vi "Main.vi"() -> ()   [LabVIEW 2013]
uses:
  source_vi/gui/type_def/device_array.ctl
  source_vi/gui/type_def/device.ctl
  source_vi/gui/type_def/general.ctl
  source_vi/gui/type_def/general_and_device.ctl
  source_vi/queues/que_enqueue_message_single.vi
  source_vi/gui/global_var.vi
panel:
  out "Application:Command Line Arguments":string[](array[string])
  out "2DArray":string[][](array[string])
  in  "config_files":string(combo) caption="Configuration file"
  out "log_bar":cluster{u8, u8}(slide) caption="Logging" scale=10.0..100.0
  out "srv_bar":cluster{u8, u8}(slide) caption="Server" scale=10.0..100.0
  in  "logging?":bool
  in  "gral_&-device":T1={"general"={"file_ext"="0.0.0.0", "TCP port"=0, "#devices"=0, "log?"=FALSE, "tcp?"=FALSE, "language"="ENG"}, "eeg_device"={"name"="", "hardware"="", "image"=path "", "path"=path "", "extra"="", "channels"=""}}
  out "eeg_device":T3
  in  "serving?":bool
  in  "acquiring?":bool
  in  "stopBars":bool
  out "acq_bar":cluster{u8, u8}(slide) caption="Acquistion" scale=10.0..100.0
  in  "log?":bool caption="Save Log"
  in  "tcp?":bool caption="Save Log"
  in  "refuse mrk?":bool
  out "images":picture[](array[picture])
  out "general":T2={"file_ext"="CSV", "TCP port"=0, "#devices"=0, "log?"=FALSE, "tcp?"=FALSE, "language"="ENG"}
  out "devices":T4
  in  "play?":bool
  out "log_box":string
  in  "stop?":bool
  in  "eeg_txtbox":string(combo) caption="Device"
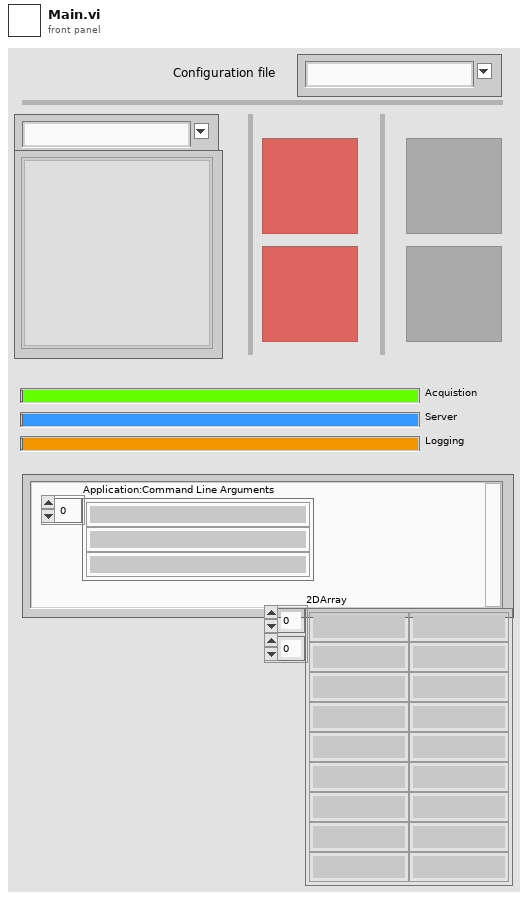
[diagram p1: front panel]
types:
  T1 = typedef "general_and_device.ctl" = cluster{"general":T2, "eeg_device":T3}
  T2 = typedef "general.ctl" = cluster{"file_ext":string, "TCP port":i32, "#devices":i32, "log?":bool, "tcp?":bool, "language":string}
  T3 = typedef "device.ctl" = cluster{"name":string, "hardware":string, "image":path, "path":path, "extra":string, "channels":string}
  T4 = typedef "device_array.ctl" = T3[]
  T5 = typedef "que_all_message_queues.ctl" = cluster{"UI":refnum<queue>, "Acquisition":refnum<queue>, "Server":refnum<queue>, "Logging":refnum<queue>}
  T6 = typedef "imagedata.ctl" = cluster{"image type":i32, "image depth":i32, "image":u8[], "mask":u8[], "colors":u32[], "Rectangle":cluster{"left":i16, "top":i16, "right":i16, "bottom":i16}}
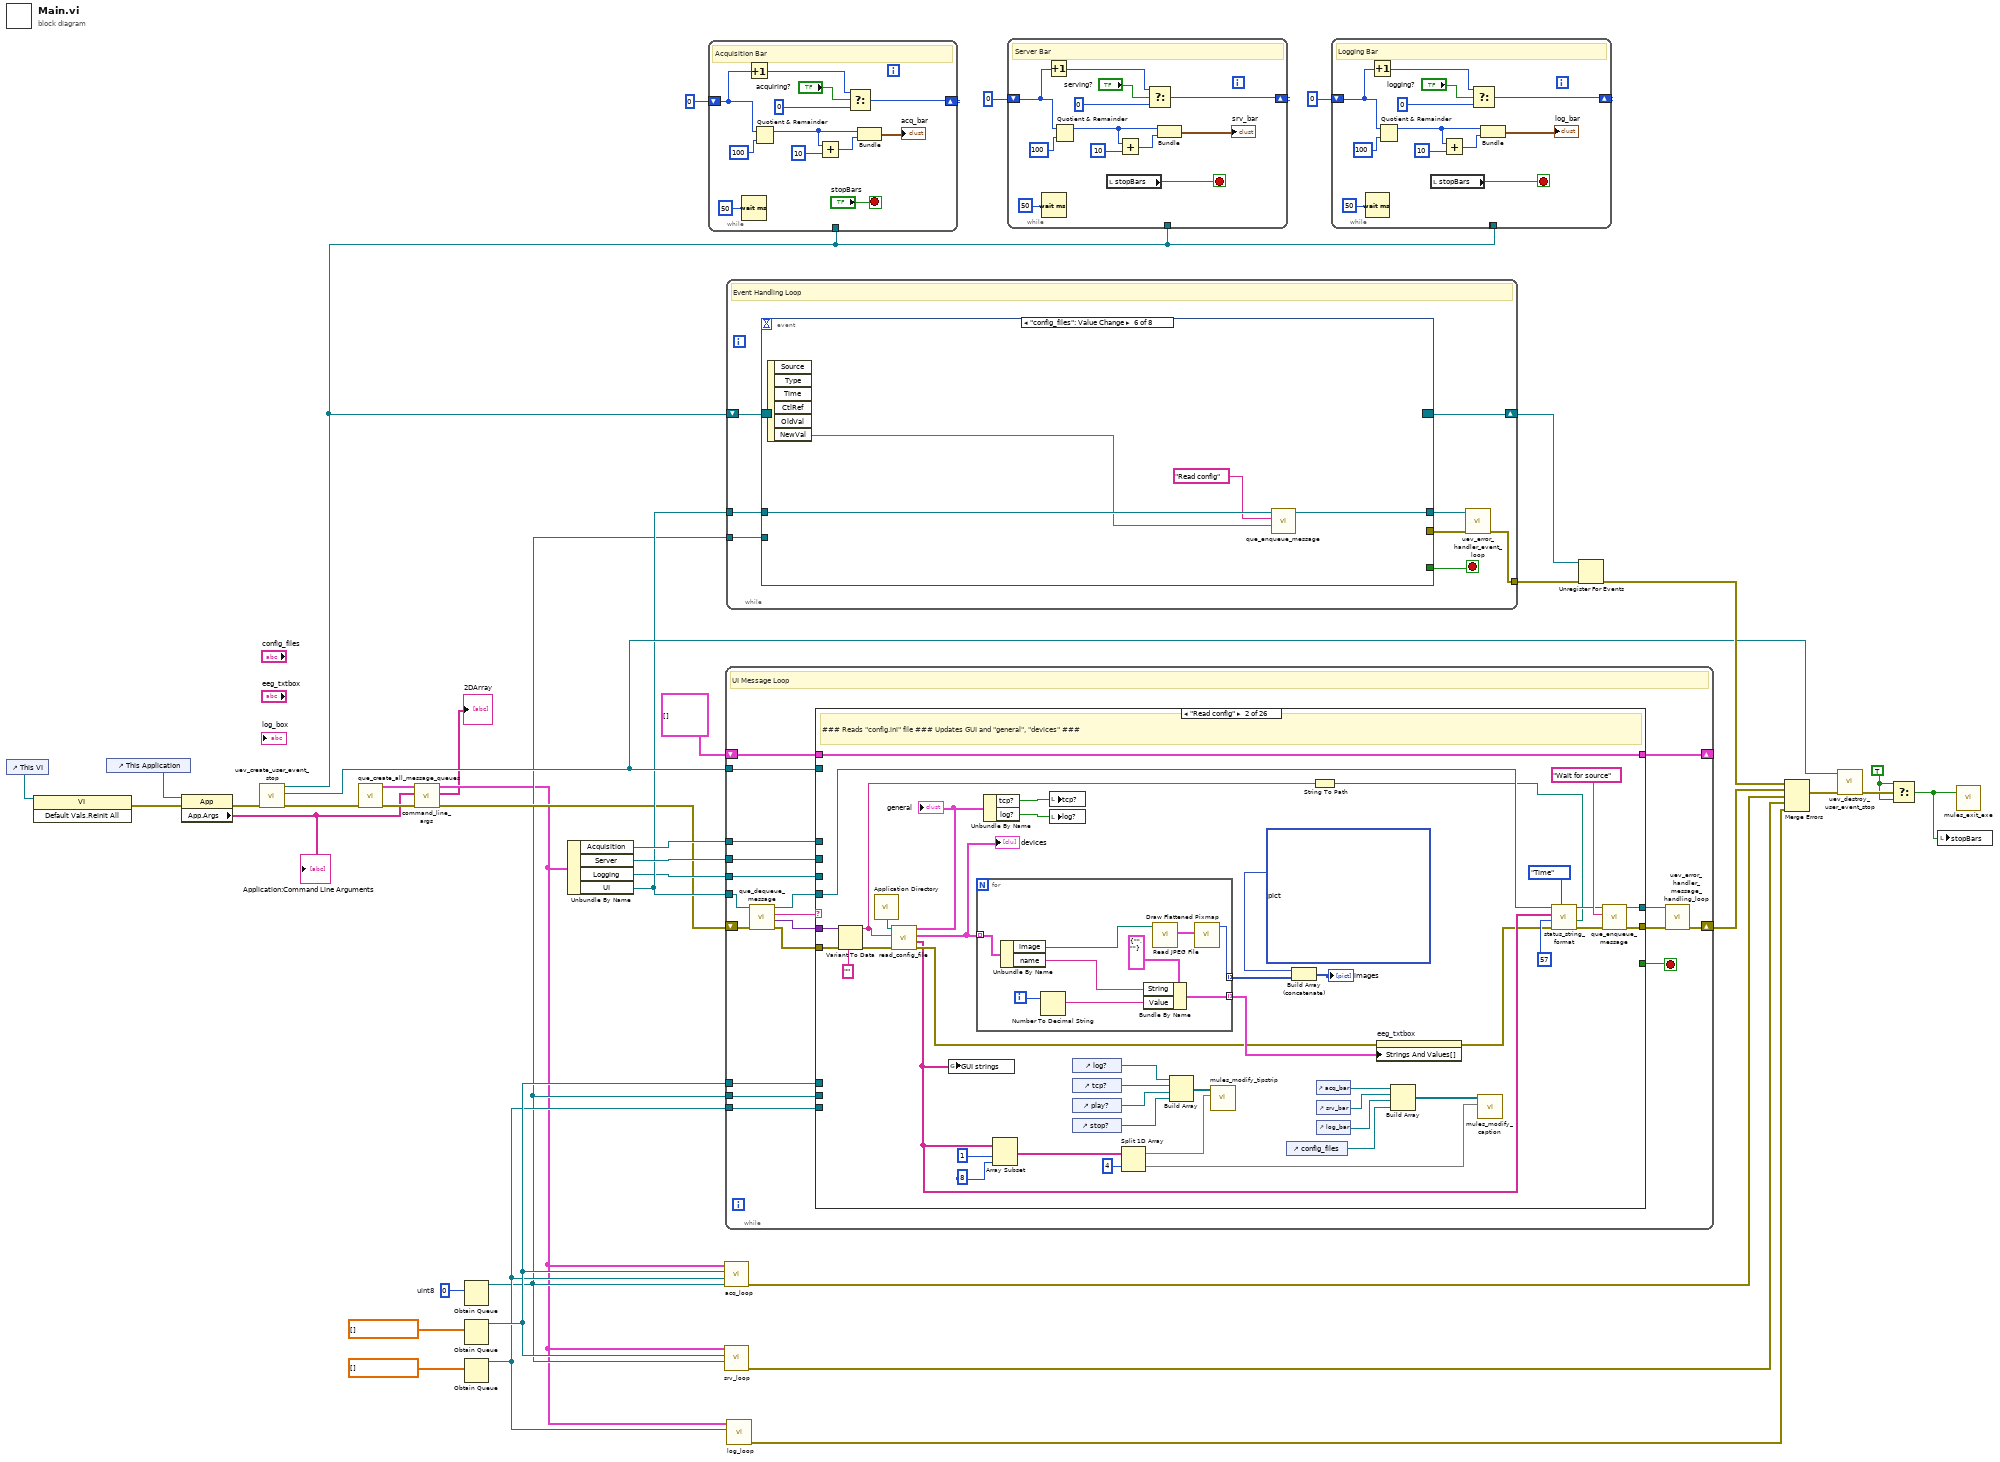
[diagram p0: block diagram]
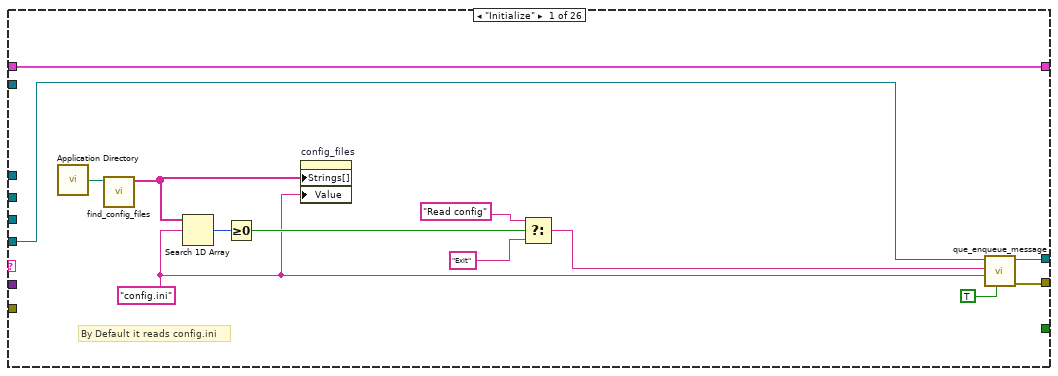
[diagram p2: hidden frame]
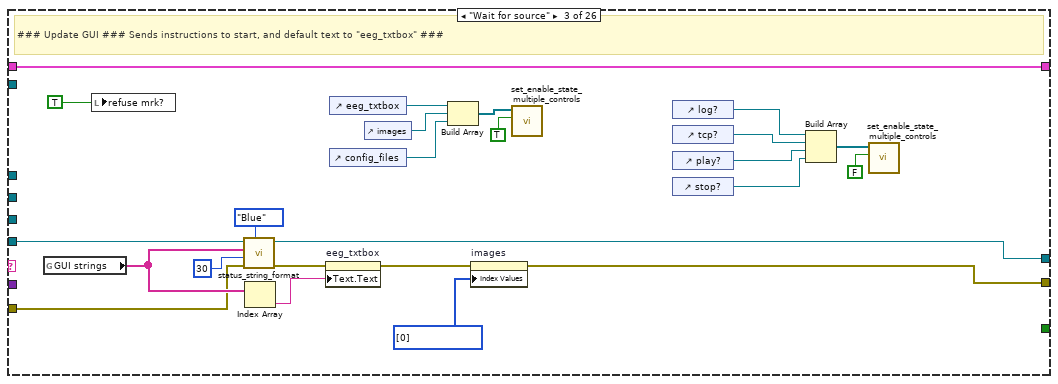
[diagram p3: hidden frame]
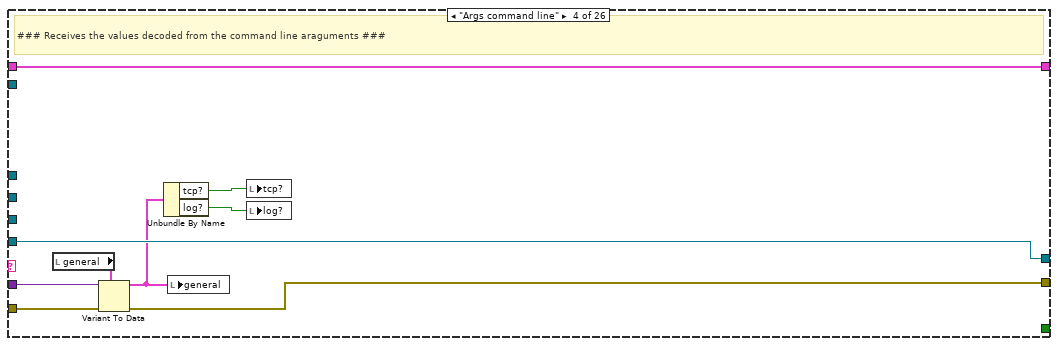
[diagram p4: hidden frame]
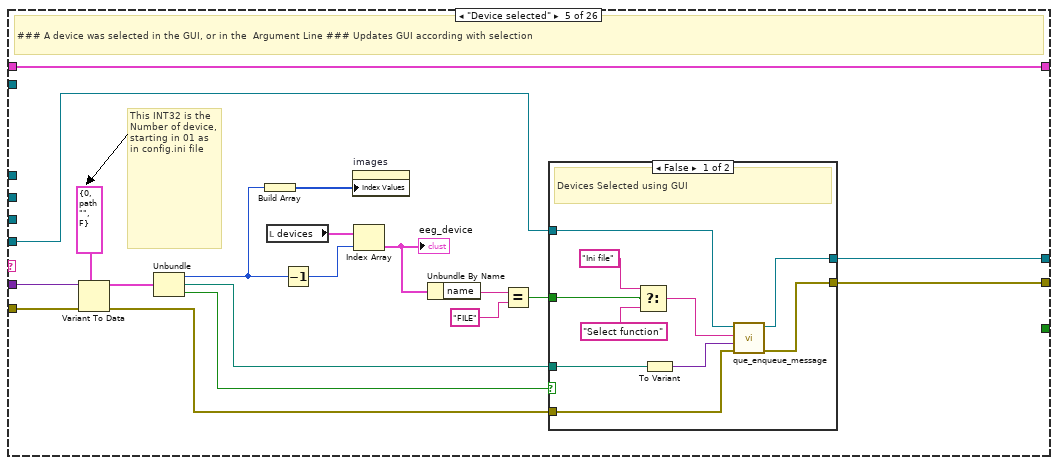
[diagram p5: hidden frame]
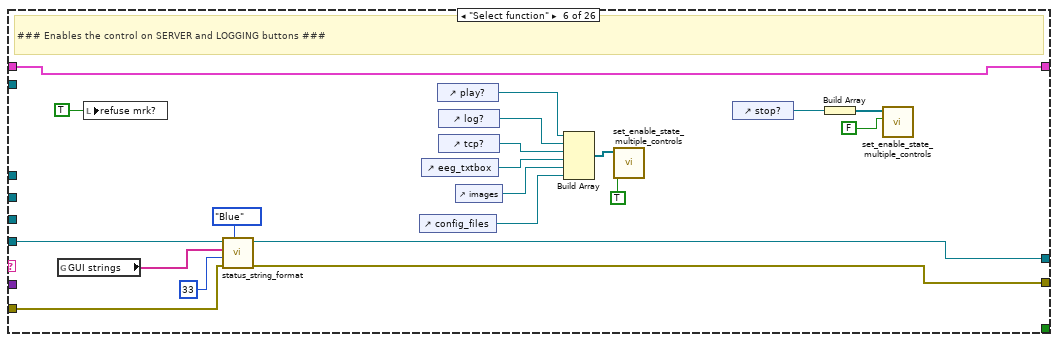
[diagram p7: hidden frame]
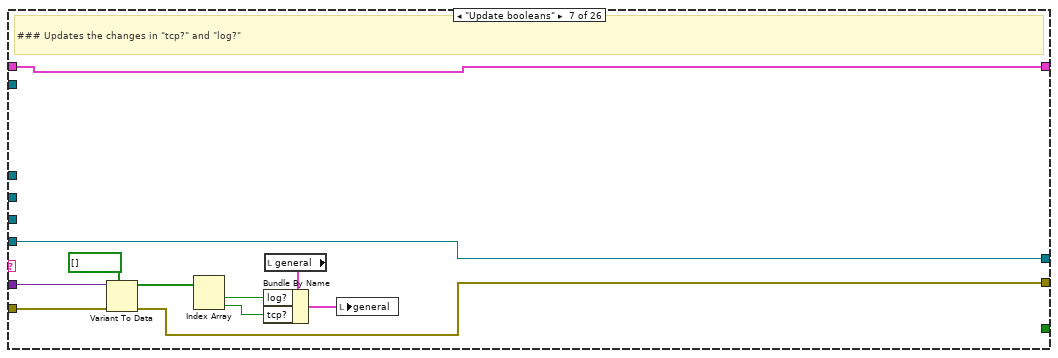
[diagram p8: hidden frame]
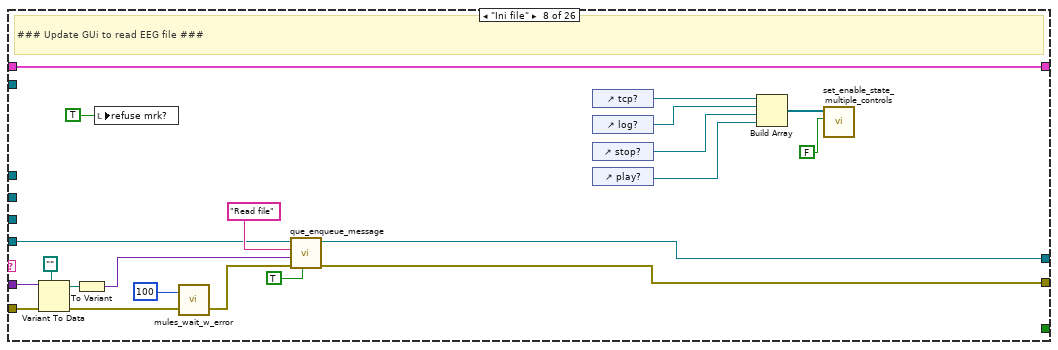
[diagram p9: hidden frame]
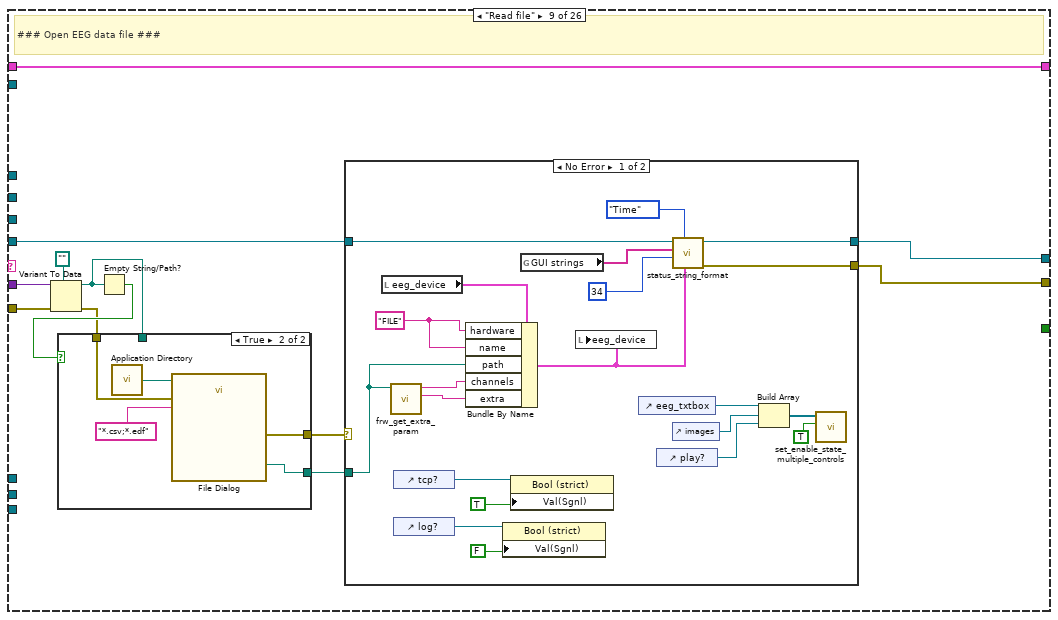
[diagram p10: hidden frame]
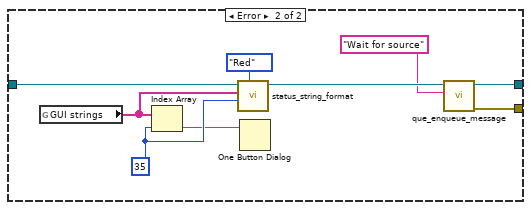
[diagram p12: hidden frame]
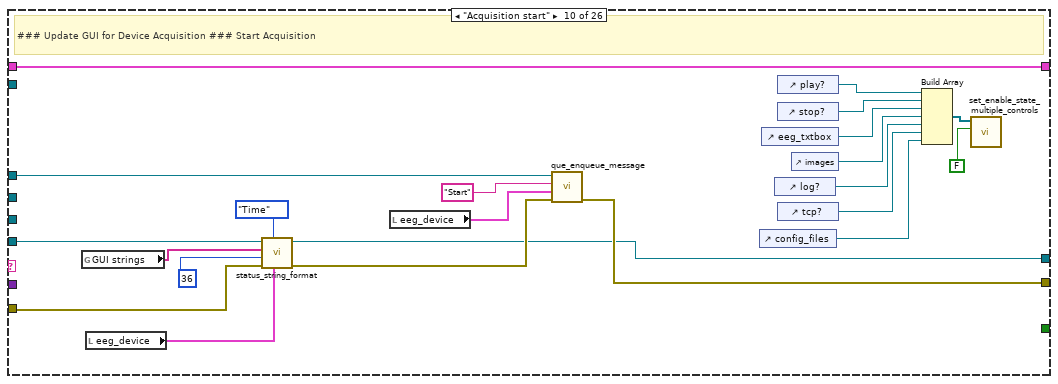
[diagram p13: hidden frame]
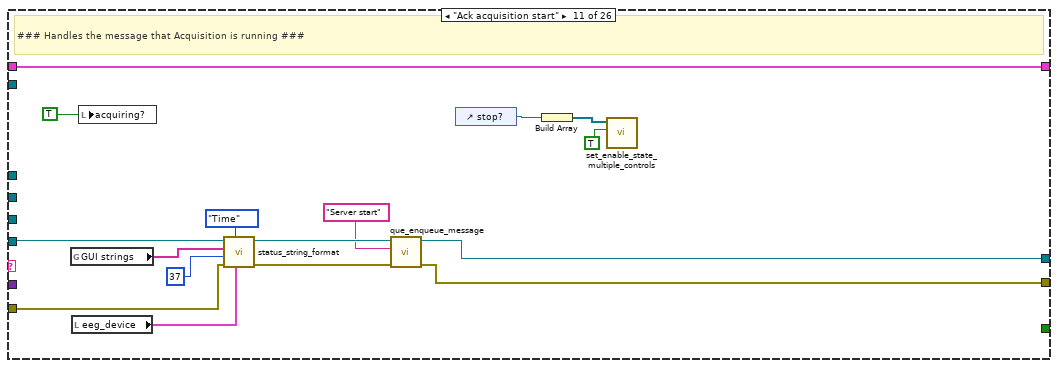
[diagram p14: hidden frame]
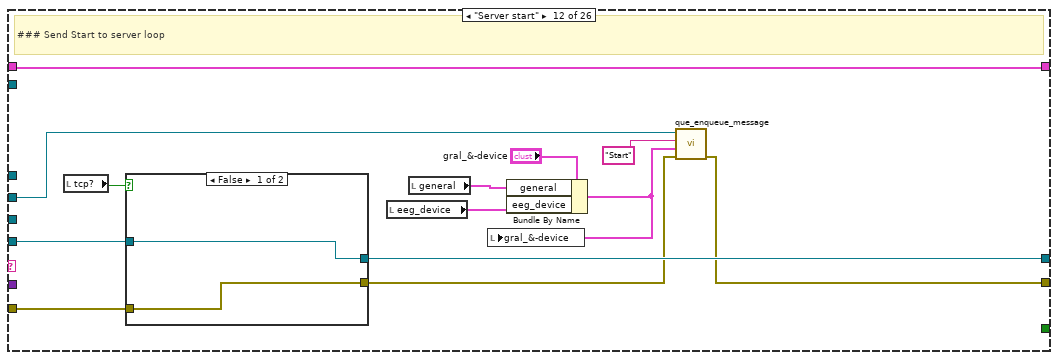
[diagram p15: hidden frame]
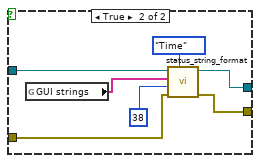
[diagram p16: hidden frame]
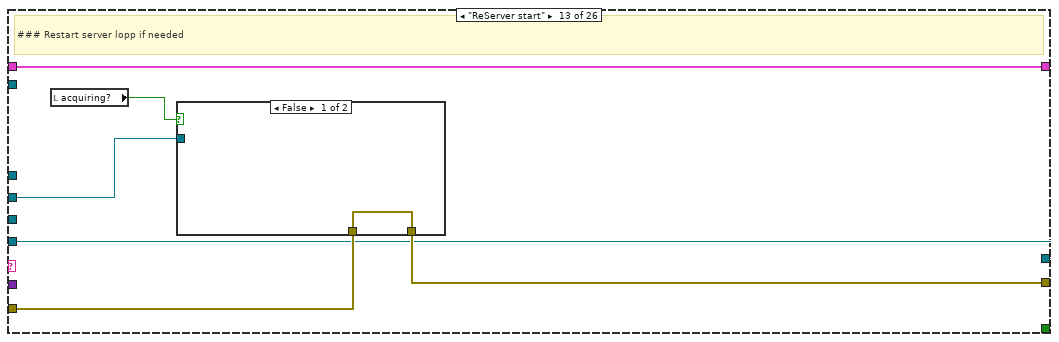
[diagram p17: hidden frame]
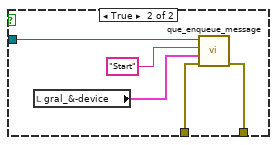
[diagram p18: hidden frame]
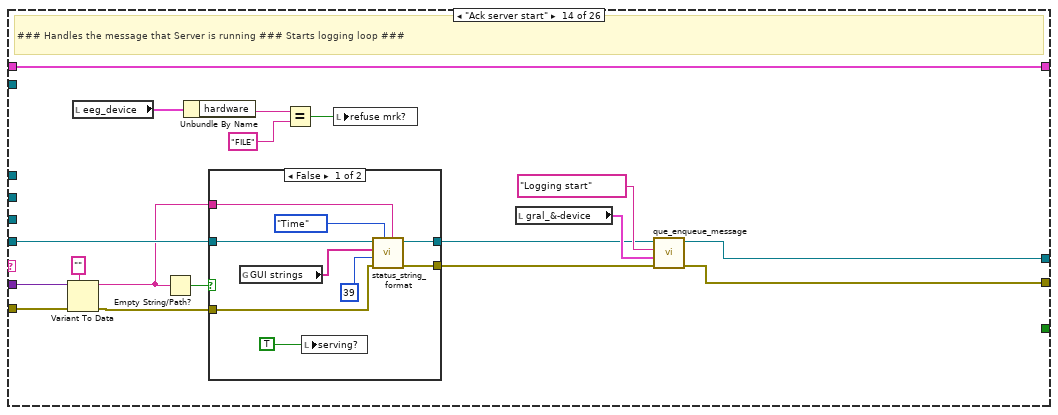
[diagram p19: hidden frame]
diagram:
  w22 = TRUE
  w29 = u8 0  # uint8
  n1 = control-ref of="This VI"() -> (w30:refnum<vi>)
  n2 = invoke class="VI" method="Default Vals.Reinit All"(reference=w30) -> (error out=w12:errorcluster)  [unwired: 2 in, 2 out]
  n3 = control-ref of="This Application"() -> (w14:refnum<vi>)
  n4 = property class="App"(reference=w14, error in=w12) -> (error out=w13:errorcluster, "App.Args"=w8:string[])  [unwired: 1 out]
  "Application:Command Line Arguments" <- w8
  n5 = call "uev_create_user_event_stop.vi"("error in (no error)"=w13) -> ("error out"=w25:errorcluster, "User Event - Stop"=w33:refnum<user-event>, "Stop Event Registration Refnum"=w6:refnum<event-registration>)  [unwired: 8 in]
  n6 = call "que_create_all_message_queues.vi"("error in (no error)"=w25) -> ("error out"=w10:errorcluster, "Message Queues out"=w9:T5)  [unwired: 9 in]
  n7 = call "command_line_args.vi"("error in (no error)"=w10, "App.Args"=w8, "Message Queues In"=w9) -> ("error out"=w11:errorcluster, "2D Array"=→"2DArray":string[][], "Message Queues Out"=w2:T5)  [unwired: 6 in]
  n8 = Obtain Queue(element data type=w29) -> (queue out=w3:refnum<queue>)  [unwired: 4 in, 2 out]
  n9 = Obtain Queue(element data type=dbl[] []) -> (queue out=w18:refnum<queue>)  [unwired: 4 in, 2 out]
  n10 = Obtain Queue(element data type=dbl[] []) -> (queue out=w4:refnum<queue>)  [unwired: 4 in, 2 out]
  n11 = Unbundle By Name(w2) -> ("Acquisition"=w32:refnum<queue>, "Server"=w31:refnum<queue>, "Logging"=w20:refnum<queue>, "UI"=w21:refnum<queue>)
  n12 = while {
    shift-right: [w42] -> _
    shift-left: 0 ("y") -> [w44]
    tunnel: w6 -> [_]
    stop <- "stopBars" stop-if-true
    # "Acquisition Bar"
    n13 = Wait (ms)(milliseconds to wait=u32 50 ("millisecond multiple")) -> ()  [unwired: 1 out]
    n14 = Increment(x=w44) -> (x+1=w43:i32)
    n15 = Quotient & Remainder(x=w44, y=100) -> (x-y*floor(x/y)=w47:i32)  [unwired: 1 out]
    n16 = Add(x=w47, y=u32 10 ("millisecond multiple")) -> (x+y=w50:u32)
    n17 = Select(t=w43, s="acquiring?", f=0 ("y")) -> (s? t:f=w42:i32)
    n18 = Bundle(w47, w50) -> (→"acq_bar":cluster{i32, u32})  [unwired: 1 in]
  }
  n19 = call "acq_loop.vi"("Marker Queue"=w3, "Log queue"=w4, "Server queue"=w18, "Message Queues"=w2) -> ("error out"=w24:errorcluster)  [unwired: 7 in]
  n20 = call "srv_loop.vi"("Marker Queue"=w3, "Server queue"=w18, "Message Queues"=w2) -> ("error out"=w19:errorcluster)  [unwired: 8 in]
  n21 = while {
    tunnel: w21 -> [w68]
    shift-right: [w56] -> w34
    shift-left: w11 -> [w69]
    tunnel: w31 -> [w63]
    tunnel: w33 -> [w62]
    tunnel: w32 -> [w61]
    tunnel: w18 -> [w54]
    tunnel: w3 -> [w59]
    shift-right: [w57] -> _
    shift-left: cluster{"String":string, "Color Box":u32}[] [] -> [w58]
    tunnel: w20 -> [w55]
    tunnel: w4 -> [w52]
    stop <- w60 stop-if-true
    # "UI Message Loop"
    n22 = call "que_dequeue_message.vi"("error in (no error)"=w69, "Message Queue"=w68) -> ("error out"=w67:errorcluster, "Message Data"=w66:variant, "Message"=w51:string, "dup Message Queue"=w65:refnum<queue>)  [unwired: 6 in]
    n23 = case shown="\"Read config\"" w51 {
      selector: w51 -> [_ _ _ _ _ _ _ _ _ _ _ _ _ _ _ _ _ _ _ _ _ _ _ _ _ w702]
      tunnel: w67 -> [_ w97 w137 w164 w168 w202 w221 w235 w252 w315 w327 w342 w363 w386 w404 w415 w438 w456 w485 w508 w532 w558 w607 w666 w693 w714]
      tunnel: w66 -> [_ w98 _ w167 w181 _ w227 w236 w255 _ _ _ _ w388 _ w416 w436 w459 w484 w512 w531 w560 w622 _ w692 _]
      tunnel: w65 -> [w77 w90 w156 w162 w178 w209 w219 w238 w262 w320 w333 w345 w361 w385 w402 w412 w444 w453 w477 w509 w528 w550 _ w663 w691 w715]
      tunnel: [w82 w93 w140 w163 w177 w201 w220 w240 w257 w310 w329 w338 w362 w379 w403 w411 w440 w461 w487 w506 w530 w548 w608 w665 w690 w703] -> w64
      tunnel: w63 -> [_ _ _ _ _ _ _ _ _ _ _ w341 w364 _ _ _ _ _ w488 _ _ _ _ _ _ w712]
      tunnel: w62 -> [_ _ _ _ _ _ _ _ _ _ _ _ _ _ _ _ _ _ _ _ _ _ _ _ _ w713]
      tunnel: w61 -> [_ _ _ _ _ _ _ _ _ w312 _ _ _ _ _ _ w442 _ _ _ _ w547 _ _ _ w711]
      tunnel: [_ _ _ _ _ _ _ _ _ _ _ _ _ _ _ _ _ _ _ _ _ _ _ _ _ TRUE ("Discard?")] -> w60
      tunnel: w54 -> [_ _ _ _ _ _ _ _ _ _ _ _ _ _ _ _ _ _ _ _ _ _ _ _ _ w708]
      tunnel: w59 -> [_ _ _ _ _ _ _ _ _ _ _ _ _ _ _ _ _ _ _ _ _ _ _ _ _ w707]
      tunnel: w58 -> [w80 w118 w139 w165 w172 w214 w222 w245 w261 w321 w323 w350 w365 w389 w401 w409 w449 w475 w490 w513 w537 w559 w620 w669 w689 w700]
      tunnel: [w80 w118 w139 w165 w172 w214 w222 w245 w261 w321 w323 w350 w365 w389 w401 w409 w449 w475 w490 w513 w537 w559 w613 w669 w689 w700] -> w57
      tunnel: w55 -> [_ _ _ _ _ _ _ _ _ _ _ _ _ _ w405 _ _ _ _ _ w524 _ _ _ _ w701]
      tunnel: [w81 w92 w136 w162 w176 w200 w219 w239 w258 w309 w328 w343 w361 w372 w402 w410 w443 w457 w478 w505 w525 w549 _ w664 w686 _] -> w53
      tunnel: w52 -> [_ _ _ _ _ _ _ _ _ _ _ _ _ _ _ _ _ _ _ _ _ _ _ _ _ w704]
      frame "Initialize" {
        w72 = "config.ini" ("Message")
        # "By Default it reads config.ini"
        n24 = call <vilib>:"Application Directory.vi"() -> ("Application Directory"=w78:path)
        n25 = call "find_config_files.vi"("path"=w78) -> ("config files_names"=w75:string[])  [unwired: 10 in]
        n26 = Search 1D Array(1D array=w75, element=w72) -> (index of element=w76:i32)  [unwired: 1 in]
        n27 = Greater Or Equal To 0?(x=w76) -> (x >= 0?=w73:bool)
        n28 = property on="config_files" class="CmbBox"("Strings[]"=w75, "Value"=w72) -> ()  [unwired: 2 in, 2 out]
        n29 = Select(t="Read config" ("Message"), s=w73, f="Exit" ("Message")) -> (s? t:f=w74:string)
        n30 = call-poly "que_enqueue_message.vi"("Priority Message? (F)"=TRUE, "Message Data"=w72, "Message"=w74, "Message Queue"=w77) -> ("error out"=w82:errorcluster, "dup Message Queue"=w81:refnum<queue>)  [unwired: 6 in]
      }
      frame "Read config" {
        # "### Reads \"config.ini\" file ### Updates GUI and \"general\", \"devices\" ###"
        n31 = Variant To Data(error in=w97, type="", Variant=w98) -> (data=w87:string, error out=w96:errorcluster)
        n32 = call <vilib>:"Application Directory.vi"() -> ("Application Directory"=w100:path)
        n33 = call "read_config_file.vi"("error in (no error)"=w96, "filename"=w87, "Application Directory"=w100) -> ("error out"=w117:errorcluster, "gui_strings"=w88:string[], "devices"=w119:T4, "gral_config"=w125:T2)  [unwired: 5 in]
        "devices" <- w119
        "general" <- w125
        n34 = global write "global_var.vi" "GUI strings"(w88) -> ()
        n35 = for {
          tunnel: w119 -> [w134] mode=indexing
          tunnel: [w132] -> w123 mode=indexing
          tunnel: [w128] -> w124 mode=indexing
          i -> [w131]
          n36 = Unbundle By Name(w134) -> ("image"=w126:path, "name"=w127:string)
          n37 = Number To Decimal String(number=w131) -> (decimal integer string=w129:string)  [unwired: 1 in]
          n38 = Bundle By Name(cluster=cluster{"String":string, "Value":string} {"String"="", "Value"=""} ("element"), "String"=w127, "Value"=w129) -> (w128:cluster{"String":string, "Value":string})
          n39 = call <vilib>:"Read JPEG File.vi"("path to JPEG file"=w126) -> ("image data"=w133:T6)  [unwired: 8 in, 2 out]
          n40 = call <vilib>:"Draw Flattened Pixmap.vi"("image data"=w133) -> ("new picture"=w132:picture)  [unwired: 8 in]
        }
        n41 = Unbundle By Name(w125) -> ("tcp?"=w121:bool, "log?"=w120:bool)
        n42 = Array Subset(array=w88, index=1, length=8) -> (w105:string[])
        n43 = local write "tcp?"(w121) -> ()
        n44 = local write "log?"(w120) -> ()
        n45 = control-ref of="log?"() -> (w114:refnum<vi>)
        n46 = control-ref of="tcp?"() -> (w113:refnum<vi>)
        n47 = control-ref of="play?"() -> (w112:refnum<vi>)
        n48 = control-ref of="stop?"() -> (w111:refnum<vi>)
        n49 = Split 1D Array(array=w105, index=4) -> (first subarray=w103:string[], second subarray=w102:string[])
        n50 = Build Array(w114, w113, w112, w111) -> (w110:refnum<vi>[])
        n51 = call "mules_modify_tipstrip.vi"("Tip Strip Array"=w103, "Controls"=w110) -> ()  [unwired: 10 in]
        n52 = control-ref of="config_files"() -> (w95:refnum<vi>)
        n53 = Build Array (concatenate)(picture bytes[110622] ("2D Picture"), w123) -> (→"images":picture[])
        n54 = String To Path(string=w87) -> (path=w86:path)
        n55 = control-ref of="acq_bar"() -> (w109:refnum<vi>)
        n56 = control-ref of="srv_bar"() -> (w108:refnum<vi>)
        n57 = control-ref of="log_bar"() -> (w107:refnum<vi>)
        n58 = property on="eeg_txtbox" class="CmbBox"(error in=w117, "Strings And Values[]"=w124) -> (error out=w83:errorcluster)  [unwired: 1 in, 1 out]
        n59 = Build Array(w109, w108, w107, w95) -> (w106:refnum<vi>[])
        n60 = call "mules_modify_caption.vi"("Tip Strip Array"=w102, "Controls"=w106) -> ()  [unwired: 10 in]
        n61 = call "status_string_format.vi"("log_file"=w86, "color"=enum16{"Black", "Blue", "Red", "Time"}."Time", "error in (no error)"=w83, "index"=57, "gui_strings"=w88, "Message Queue"=w90) -> ("error out"=w89:errorcluster, "dup Message Queue"=w91:refnum<queue>)  [unwired: 4 in]
        n62 = call-poly "que_enqueue_message.vi"("error in (no error)"=w89, "Message"="Wait for source", "Message Queue"=w91) -> ("error out"=w93:errorcluster, "dup Message Queue"=w92:refnum<queue>)  [unwired: 7 in]
      }
      frame "Wait for source" {
        # "### Update GUI ### Sends instructions to start, and default text to \"eeg_txtbox\" ###"
        n63 = global read "global_var.vi" "GUI strings"() -> (w138:string[])
        n64 = local write "refuse mrk?"(TRUE) -> ()
        n65 = call "status_string_format.vi"("color"=enum16{"Black", "Blue", "Red", "Time"}."Blue", "error in (no error)"=w137, "index"=30, "gui_strings"=w138, "Message Queue"=w156) -> ("error out"=w152:errorcluster, "dup Message Queue"=w136:refnum<queue>)  [unwired: 5 in]
        n66 = Index Array(array=w138) -> (element=w153:string)  [unwired: 1 in]
        n67 = property on="eeg_txtbox" class="CmbBox"(error in=w152, "Text.Text"=w153) -> (error out=w155:errorcluster)  [unwired: 1 in, 1 out]
        n68 = control-ref of="eeg_txtbox"() -> (w144:refnum<vi>)
        n69 = control-ref of="config_files"() -> (w135:refnum<vi>)
        n70 = control-ref of="images"() -> (w143:refnum<vi>)
        n71 = Build Array(w144, w143, w135) -> (w141:refnum<vi>[])
        n72 = property on="images" class="Arr (strict)"(error in=w155, "Index Values"=u32[] [0]) -> (error out=w140:errorcluster)  [unwired: 1 in, 1 out]
        n73 = call "set_enable_state_multiple_controls.vi"("Enable?"=TRUE, "Controls"=w141) -> ()  [unwired: 10 in]
        n74 = control-ref of="log?"() -> (w145:refnum<vi>)
        n75 = control-ref of="tcp?"() -> (w146:refnum<vi>)
        n76 = control-ref of="play?"() -> (w147:refnum<vi>)
        n77 = control-ref of="stop?"() -> (w148:refnum<vi>)
        n78 = Build Array(w145, w146, w147, w148) -> (w151:refnum<vi>[])
        n79 = call "set_enable_state_multiple_controls.vi"("Enable?"=FALSE, "Controls"=w151) -> ()  [unwired: 10 in]
      }
      frame "Args command line" {
        # "### Receives the values decoded from the command line araguments ###"
        n80 = local read "general"() -> (w166:T2)
        n81 = Variant To Data(error in=w164, type=w166, Variant=w167) -> (data=w159:T2, error out=w163:errorcluster)
        n82 = Unbundle By Name(w159) -> ("tcp?"=w161:bool, "log?"=w160:bool)
        n83 = local write "general"(w159) -> ()
        n84 = local write "tcp?"(w161) -> ()
        n85 = local write "log?"(w160) -> ()
      }
      frame "Device selected" {
        # "This INT32 is the Number of device, starting in 01 as in config.ini file"
        # "### A device was selected in the GUI, or in the  Argument Line ### Updates GUI according with selection"
        n86 = Variant To Data(error in=w168, type=cluster{i32, path, bool} {0, path "", FALSE} ("output cluster"), Variant=w181) -> (data=w175:cluster{i32, path, bool}, error out=w169:errorcluster)
        n87 = Unbundle(w175) -> (w174:i32, w173:path, w170:bool)
        n88 = Build Array(w174) -> (w180:i32[])
        n89 = local read "devices"() -> (w182:T4)
        n90 = Decrement(x=w174) -> (x-1=w179:i32)
        n91 = property on="images" class="Arr (strict)"("Index Values"=w180) -> ()  [unwired: 2 in, 2 out]
        n92 = Index Array(array=w182, index=w179) -> (element=w183:T3)
        "eeg_device" <- w183
        n93 = Unbundle By Name(w183) -> ("name"=w184:string)
        n94 = Equal?(x=w184, y="FILE" ("Message")) -> (x = y?=w186:bool)
        n95 = case shown="False" w170 {
          tunnel: w186 -> [w193 _]
          tunnel: w178 -> [w192 w198]
          tunnel: [w191 w197] -> w177
          tunnel: [w190 w198] -> w176
          tunnel: w173 -> [w189 _]
          tunnel: w169 -> [w187 w197]
          frame False {
            # "Devices Selected using GUI"
            n96 = Select(t="Ini file" ("Message"), s=w193, f="Select function" ("Message")) -> (s? t:f=w196:string)
            n97 = To Variant(anything=w189) -> (Variant=w188:variant)
            n98 = call-poly "que_enqueue_message.vi"("error in (no error)"=w187, "Message Data"=w188, "Message"=w196, "Message Queue"=w192) -> ("error out"=w191:errorcluster, "dup Message Queue"=w190:refnum<queue>)  [unwired: 6 in]
          }
          frame True {
            # "Device Selected in Argument Line"
          }
        }
      }
      frame "Select function" {
        # "### Enables the control on SERVER and LOGGING buttons ###"
        n99 = global read "global_var.vi" "GUI strings"() -> (w208:string[])
        n100 = local write "refuse mrk?"(TRUE) -> ()
        n101 = call "status_string_format.vi"("color"=enum16{"Black", "Blue", "Red", "Time"}."Blue", "error in (no error)"=w202, "index"=33, "gui_strings"=w208, "Message Queue"=w209) -> ("error out"=w201:errorcluster, "dup Message Queue"=w200:refnum<queue>)  [unwired: 5 in]
        n102 = control-ref of="config_files"() -> (w199:refnum<vi>)
        n103 = control-ref of="eeg_txtbox"() -> (w211:refnum<vi>)
        n104 = control-ref of="play?"() -> (w203:refnum<vi>)
        n105 = control-ref of="log?"() -> (w204:refnum<vi>)
        n106 = control-ref of="tcp?"() -> (w205:refnum<vi>)
        n107 = control-ref of="images"() -> (w210:refnum<vi>)
        n108 = Build Array(w203, w204, w205, w211, w210, w199) -> (w213:refnum<vi>[])
        n109 = call "set_enable_state_multiple_controls.vi"("Enable?"=TRUE, "Controls"=w213) -> ()  [unwired: 10 in]
        n110 = control-ref of="stop?"() -> (w218:refnum<vi>)
        n111 = Build Array(w218) -> (w217:refnum<vi>[])
        n112 = call "set_enable_state_multiple_controls.vi"("Enable?"=FALSE, "Controls"=w217) -> ()  [unwired: 10 in]
      }
      frame "Update booleans" {
        # "### Updates the changes in \"tcp?\" and \"log?\""
        n113 = Variant To Data(error in=w221, type=bool[] [], Variant=w227) -> (data=w225:bool[], error out=w220:errorcluster)
        n114 = Index Array(array=w225) -> (element #1=w224:bool, element #2=w223:bool)  [unwired: 2 in]
        n115 = local read "general"() -> (w228:T2)
        n116 = Bundle By Name(cluster=w228, "log?"=w224, "tcp?"=w223) -> (w229:T2)
        n117 = local write "general"(w229) -> ()
      }
      frame "Ini file" {
        # "### Update GUi to read EEG file ###"
        n118 = Variant To Data(error in=w235, type=path "", Variant=w236) -> (data=w232:path, error out=w234:errorcluster)
        n119 = To Variant(anything=w232) -> (Variant=w231:variant)
        n120 = local write "refuse mrk?"(TRUE) -> ()
        n121 = call "mules_wait_w_error.vi"("error in (no error)"=w234, "milliseconds to wait"=u32 100) -> ("error out"=w242:errorcluster)  [unwired: 1 in]
        n122 = call-poly "que_enqueue_message.vi"("Priority Message? (F)"=TRUE, "error in (no error)"=w242, "Message Data"=w231, "Message"="Read file", "Message Queue"=w238) -> ("error out"=w240:errorcluster, "dup Message Queue"=w239:refnum<queue>)  [unwired: 5 in]
        n123 = control-ref of="tcp?"() -> (w237:refnum<vi>)
        n124 = control-ref of="log?"() -> (w244:refnum<vi>)
        n125 = control-ref of="stop?"() -> (w250:refnum<vi>)
        n126 = control-ref of="play?"() -> (w249:refnum<vi>)
        n127 = Build Array(w237, w244, w250, w249) -> (w248:refnum<vi>[])
        n128 = call "set_enable_state_multiple_controls.vi"("Enable?"=FALSE, "Controls"=w248) -> ()  [unwired: 10 in]
      }
      frame "Read file" {
        # "### Open EEG data file ###"
        n129 = Variant To Data(error in=w252, type=path "", Variant=w255) -> (data=w253:path, error out=w251:errorcluster)
        n130 = Empty String/Path?(string/path=w253) -> (empty?=w254:bool)
        n131 = case shown="True" w254 {
          tunnel: [w263 w269] -> w260
          tunnel: [w264 w268] -> w259
          tunnel: w253 -> [w264 _]
          tunnel: w251 -> [w263 w267]
          frame False {
          }
          frame True {
            n132 = call <vilib>:"Application Directory.vi"() -> ("Application Directory"=w265:path)
            n133 = call "File Dialog"("start path"=w265, "error in"=w267, "pattern (all files)"="*.csv;*.edf") -> ("selected path"=w268:path, "error out"=w269:errorcluster)  [unwired: 9 in, 2 out]
          }
        }
        n134 = case shown="No Error" w260 {
          tunnel: w262 -> [w286 w299]
          tunnel: w259 -> [w283 _]
          tunnel: [w287 w294] -> w258
          tunnel: [w279 w292] -> w257
          frame No Error {
            w280 = "FILE" ("Message")
            n135 = local read "eeg_device"() -> (w290:T3)
            n136 = call "frw_get_extra_param.vi"("Path"=w283) -> ("extra_string"=w281:string, "channels_str"=w282:string)  [unwired: 9 in]
            n137 = control-ref of="tcp?"() -> (w270:refnum<vi>)
            n138 = control-ref of="log?"() -> (w273:refnum<vi>)
            n139 = Bundle By Name(cluster=w290, "hardware"=w280, "name"=w280, "path"=w283, "channels"=w282, "extra"=w281) -> (w285:T3)
            n140 = property class="Bool (strict)"(reference=w273, "Val(Sgnl)"=FALSE ("Value (Signaling)")) -> ()  [unwired: 1 in, 2 out]
            n141 = property class="Bool (strict)"(reference=w270, "Val(Sgnl)"=TRUE ("Value (Signaling)")) -> ()  [unwired: 1 in, 2 out]
            n142 = global read "global_var.vi" "GUI strings"() -> (w289:string[])
            n143 = local write "eeg_device"(w285) -> ()
            n144 = control-ref of="eeg_txtbox"() -> (w275:refnum<vi>)
            n145 = control-ref of="play?"() -> (w277:refnum<vi>)
            n146 = call "status_string_format.vi"("eeg_device"=w285, "color"=enum16{"Black", "Blue", "Red", "Time"}."Time", "index"=34, "gui_strings"=w289, "Message Queue"=w286) -> ("error out"=w279:errorcluster, "dup Message Queue"=w287:refnum<queue>)  [unwired: 5 in]
            n147 = control-ref of="images"() -> (w274:refnum<vi>)
            n148 = Build Array(w275, w274, w277) -> (w276:refnum<vi>[])
            n149 = call "set_enable_state_multiple_controls.vi"("Enable?"=TRUE, "Controls"=w276) -> ()  [unwired: 10 in]
          }
          frame Error {
            w297 = 35 ("index")
            n150 = global read "global_var.vi" "GUI strings"() -> (w298:string[])
            n151 = Index Array(array=w298, index=w297) -> (element=w291:string)
            n152 = call "status_string_format.vi"("color"=enum16{"Black", "Blue", "Red", "Time"}."Red", "index"=w297, "gui_strings"=w298, "Message Queue"=w299) -> ("dup Message Queue"=w295:refnum<queue>)  [unwired: 6 in, 1 out]
            n153 = One Button Dialog(message=w291) -> ()  [unwired: 1 in, 1 out]
            n154 = call-poly "que_enqueue_message.vi"("Message"="Wait for source", "Message Queue"=w295) -> ("error out"=w292:errorcluster, "dup Message Queue"=w294:refnum<queue>)  [unwired: 8 in]
          }
        }
      }
      frame "Acquisition start" {
        # "### Update GUI for Device Acquisition ### Start Acquisition"
        n155 = global read "global_var.vi" "GUI strings"() -> (w319:string[])
        n156 = local read "eeg_device"() -> (w316:T3)
        n157 = call "status_string_format.vi"("eeg_device"=w316, "color"=enum16{"Black", "Blue", "Red", "Time"}."Time", "error in (no error)"=w315, "index"=36, "gui_strings"=w319, "Message Queue"=w320) -> ("error out"=w311:errorcluster, "dup Message Queue"=w309:refnum<queue>)  [unwired: 4 in]
        n158 = local read "eeg_device"() -> (w313:T3)
        n159 = call-poly "que_enqueue_message.vi"("error in (no error)"=w311, "Message Data"=w313, "Message"="Start", "Message Queue"=w312) -> ("error out"=w310:errorcluster)  [unwired: 6 in, 1 out]
        n160 = control-ref of="config_files"() -> (w300:refnum<vi>)
        n161 = control-ref of="eeg_txtbox"() -> (w304:refnum<vi>)
        n162 = control-ref of="log?"() -> (w302:refnum<vi>)
        n163 = control-ref of="play?"() -> (w308:refnum<vi>)
        n164 = control-ref of="stop?"() -> (w307:refnum<vi>)
        n165 = control-ref of="tcp?"() -> (w301:refnum<vi>)
        n166 = control-ref of="images"() -> (w303:refnum<vi>)
        n167 = Build Array(w308, w307, w304, w303, w302, w301, w300) -> (w306:refnum<vi>[])
        n168 = call "set_enable_state_multiple_controls.vi"("Enable?"=FALSE, "Controls"=w306) -> ()  [unwired: 10 in]
      }
      frame "Ack acquisition start" {
        # "### Handles the message that Acquisition is running ###"
        n169 = global read "global_var.vi" "GUI strings"() -> (w337:string[])
        n170 = local read "eeg_device"() -> (w334:T3)
        n171 = local write "acquiring?"(TRUE ("runBar1?")) -> ()
        n172 = call "status_string_format.vi"("eeg_device"=w334, "color"=enum16{"Black", "Blue", "Red", "Time"}."Time", "error in (no error)"=w327, "index"=37, "gui_strings"=w337, "Message Queue"=w333) -> ("error out"=w330:errorcluster, "dup Message Queue"=w332:refnum<queue>)  [unwired: 4 in]
        n173 = call-poly "que_enqueue_message.vi"("error in (no error)"=w330, "Message"="Server start", "Message Queue"=w332) -> ("error out"=w329:errorcluster, "dup Message Queue"=w328:refnum<queue>)  [unwired: 7 in]
        n174 = control-ref of="stop?"() -> (w326:refnum<vi>)
        n175 = Build Array(w326) -> (w325:refnum<vi>[])
        n176 = call "set_enable_state_multiple_controls.vi"("Enable?"=TRUE, "Controls"=w325) -> ()  [unwired: 10 in]
      }
      frame "Server start" {
        # "### Send Start to server loop"
        n177 = local read "tcp?"() -> (w344:bool)
        n178 = case shown="False" w344 {
          tunnel: w345 -> [w351 w356]
          tunnel: w342 -> [w352 w355]
          tunnel: [w351 w354] -> w343
          tunnel: [w352 w353] -> w339
          frame False {
          }
          frame True {
            n179 = global read "global_var.vi" "GUI strings"() -> (w358:string[])
            n180 = call "status_string_format.vi"("color"=enum16{"Black", "Blue", "Red", "Time"}."Time", "error in (no error)"=w355, "index"=38, "gui_strings"=w358, "Message Queue"=w356) -> ("error out"=w353:errorcluster, "dup Message Queue"=w354:refnum<queue>)  [unwired: 5 in]
          }
        }
        n181 = local read "eeg_device"() -> (w346:T3)
        n182 = local read "general"() -> (w347:T2)
        n183 = Bundle By Name(cluster="gral_&-device", "general"=w347, "eeg_device"=w346) -> (w340:T1)
        n184 = local write "gral_&-device"(w340) -> ()
        n185 = call-poly "que_enqueue_message.vi"("error in (no error)"=w339, "Message Data"=w340, "Message"="Start", "Message Queue"=w341) -> ("error out"=w338:errorcluster)  [unwired: 6 in, 1 out]
      }
      frame "ReServer start" {
        # "### Restart server lopp if needed"
        n186 = local read "acquiring?"() -> (w360:bool)
        n187 = case shown="False" w360 {
          tunnel: w364 -> [_ w370]
          tunnel: w363 -> [w366 w368]
          tunnel: [w366 w367] -> w362
          frame False {
          }
          frame True {
            n188 = local read "gral_&-device"() -> (w369:T1)
            n189 = call-poly "que_enqueue_message.vi"("error in (no error)"=w368, "Message Data"=w369, "Message"="Start", "Message Queue"=w370) -> ("error out"=w367:errorcluster)  [unwired: 6 in, 1 out]
          }
        }
      }
      frame "Ack server start" {
        # "### Handles the message that Server is running ### Starts logging loop ###"
        n190 = Variant To Data(error in=w386, type="" ("String"), Variant=w388) -> (data=w381:string, error out=w378:errorcluster)
        n191 = local read "eeg_device"() -> (w377:T3)
        n192 = Empty String/Path?(string/path=w381) -> (empty?=w382:bool)
        n193 = Unbundle By Name(w377) -> ("hardware"=w376:string)
        n194 = case shown="False" w382 {
          tunnel: w385 -> [w398 w399]
          tunnel: w381 -> [w394 _]
          tunnel: [w393 w400] -> w380
          tunnel: w378 -> [w392 w400]
          tunnel: [w391 w399] -> w373
          frame False {
            n195 = global read "global_var.vi" "GUI strings"() -> (w397:string[])
            n196 = local write "serving?"(TRUE ("runBar1?")) -> ()
            n197 = call "status_string_format.vi"("ip"=w394, "color"=enum16{"Black", "Blue", "Red", "Time"}."Time", "error in (no error)"=w392, "index"=39, "gui_strings"=w397, "Message Queue"=w398) -> ("error out"=w393:errorcluster, "dup Message Queue"=w391:refnum<queue>)  [unwired: 4 in]
          }
          frame True {
          }
        }
        n198 = Equal?(x=w376, y="FILE") -> (x = y?=w374:bool)
        n199 = local write "refuse mrk?"(w374) -> ()
        n200 = local read "gral_&-device"() -> (w383:T1)
        n201 = call-poly "que_enqueue_message.vi"("error in (no error)"=w380, "Message Data"=w383, "Message"="Logging start", "Message Queue"=w373) -> ("error out"=w379:errorcluster, "dup Message Queue"=w372:refnum<queue>)  [unwired: 6 in]
      }
      frame "Logging start" {
        n202 = local read "gral_&-device"() -> (w406:T1)
        n203 = call-poly "que_enqueue_message.vi"("error in (no error)"=w404, "Message Data"=w406, "Message"="Start", "Message Queue"=w405) -> ("error out"=w403:errorcluster)  [unwired: 6 in, 1 out]
      }
      frame "Ack logging start" {
        n204 = Variant To Data(error in=w415, type=path[] [], Variant=w416) -> (data=w414:path[], error out=w413:errorcluster)
        n205 = for {
          tunnel: w414 -> [w421] mode=indexing
          tunnel: w412 -> [w422]
          tunnel: [w420] -> w411
          tunnel: w413 -> [w419]
          tunnel: [w418] -> w410
          n206 = Empty String/Path?(string/path=w421) -> (empty?=w423:bool)
          n207 = case shown="False" w423 {
            tunnel: w422 -> [w430 w432]
            tunnel: w421 -> [w429 _]
            tunnel: [w426 w433] -> w420
            tunnel: w419 -> [w425 w433]
            tunnel: [w424 w432] -> w418
            frame False {
              n208 = global read "global_var.vi" "GUI strings"() -> (w431:string[])
              n209 = call "status_string_format.vi"("log_file"=w429, "color"=enum16{"Black", "Blue", "Red", "Time"}."Time", "error in (no error)"=w425, "index"=53, "gui_strings"=w431, "Message Queue"=w430) -> ("error out"=w426:errorcluster, "dup Message Queue"=w424:refnum<queue>)  [unwired: 4 in]
            }
            frame True {
            }
          }
        }
        n210 = local read "log?"() -> (w408:bool)
        n211 = local write "logging?"(w408) -> ()
      }
      frame "Acquisition stop" {
        w439 = 0  # int32
        # "### Stops Acquisition ###"
        n212 = Variant To Data(error in=w438, type=w439, Variant=w436) -> (data=w434:i32, error out=w437:errorcluster)
        n213 = To Variant(anything=w434) -> (Variant=w435:variant)
        n214 = global read "global_var.vi" "GUI strings"() -> (w448:string[])
        n215 = local read "eeg_device"() -> (w445:T3)
        n216 = call "status_string_format.vi"("eeg_device"=w445, "color"=enum16{"Black", "Blue", "Red", "Time"}."Time", "error in (no error)"=w437, "index"=45, "gui_strings"=w448, "Message Queue"=w444) -> ("error out"=w441:errorcluster, "dup Message Queue"=w443:refnum<queue>)  [unwired: 4 in]
        n217 = call-poly "que_enqueue_message.vi"("error in (no error)"=w441, "Message Data"=w435, "Message"="Stop", "Message Queue"=w442) -> ("error out"=w440:errorcluster)  [unwired: 6 in, 1 out]
      }
      frame "Ack acquisition stop" {
        w458 = 0  # int32
        # "### Handles the message that Acquisition is stopped ###"
        n218 = Variant To Data(error in=w456, type=w458, Variant=w459) -> (data=w455:i32, error out=w452:errorcluster)
        n219 = local write "acquiring?"(FALSE ("runBar1?")) -> ()
        n220 = global read "global_var.vi" "GUI strings"() -> (w464:string[])
        n221 = local read "eeg_device"() -> (w466:T3)
        n222 = call "status_string_format.vi"("eeg_device"=w466, "color"=enum16{"Black", "Blue", "Red", "Time"}."Time", "error in (no error)"=w452, "index"=46, "gui_strings"=w464, "Message Queue"=w453) -> ("dup Message Queue"=w454:refnum<queue>)  [unwired: 4 in, 1 out]
        n223 = To Variant(anything=w455) -> (Variant=w460:variant)
        n224 = call-poly "que_enqueue_message.vi"("Message Data"=w460, "Message"="Server stop", "Message Queue"=w454) -> ("error out"=w461:errorcluster, "dup Message Queue"=w457:refnum<queue>)  [unwired: 7 in]
        n225 = control-ref of="config_files"() -> (w451:refnum<vi>)
        n226 = control-ref of="eeg_txtbox"() -> (w470:refnum<vi>)
        n227 = control-ref of="log?"() -> (w468:refnum<vi>)
        n228 = control-ref of="play?"() -> (w474:refnum<vi>)
        n229 = control-ref of="stop?"() -> (w473:refnum<vi>)
        n230 = control-ref of="tcp?"() -> (w467:refnum<vi>)
        n231 = control-ref of="images"() -> (w469:refnum<vi>)
        n232 = Build Array(w451, w474, w473, w470, w469, w468, w467) -> (w472:refnum<vi>[])
        n233 = call "set_enable_state_multiple_controls.vi"("Enable?"=FALSE, "Controls"=w472) -> ()  [unwired: 10 in]
      }
      frame "Server stop" {
        w486 = 0  # int32
        n234 = Variant To Data(error in=w485, type=w486, Variant=w484) -> (data=w482:i32, error out=w480:errorcluster)
        n235 = local read "tcp?"() -> (w481:bool)
        n236 = case shown="True" w481 {
          tunnel: w477 -> [w492 w496]
          tunnel: [w491 w495] -> w479
          tunnel: [w492 w494] -> w478
          tunnel: w480 -> [w491 w493]
          frame False {
          }
          frame True {
            n237 = global read "global_var.vi" "GUI strings"() -> (w497:string[])
            n238 = call "status_string_format.vi"("color"=enum16{"Black", "Blue", "Red", "Time"}."Time", "error in (no error)"=w493, "index"=54, "gui_strings"=w497, "Message Queue"=w496) -> ("error out"=w495:errorcluster, "dup Message Queue"=w494:refnum<queue>)  [unwired: 5 in]
          }
        }
        n239 = To Variant(anything=w482) -> (Variant=w483:variant)
        n240 = call-poly "que_enqueue_message.vi"("error in (no error)"=w479, "Message Data"=w483, "Message"="Stop", "Message Queue"=w488) -> ("error out"=w487:errorcluster)  [unwired: 6 in, 1 out]
      }
      frame "Ack server stop" {
        w511 = 0  # Int32
        # "### Handles the message that Server is stopped ###"
        n241 = Variant To Data(error in=w508, type=w511, Variant=w512) -> (data=w510:i32, error out=w507:errorcluster)
        n242 = local write "serving?"(FALSE ("runBar1?")) -> ()
        n243 = local read "tcp?"() -> (w503:bool)
        n244 = case shown="True" w503 {
          tunnel: w509 -> [w516 w520]
          tunnel: [w515 w519] -> w501
          tunnel: [w516 w518] -> w502
          tunnel: w507 -> [w515 w517]
          frame False {
          }
          frame True {
            n245 = global read "global_var.vi" "GUI strings"() -> (w521:string[])
            n246 = call "status_string_format.vi"("color"=enum16{"Black", "Blue", "Red", "Time"}."Time", "error in (no error)"=w517, "index"=40, "gui_strings"=w521, "Message Queue"=w520) -> ("error out"=w519:errorcluster, "dup Message Queue"=w518:refnum<queue>)  [unwired: 5 in]
          }
        }
        n247 = To Variant(anything=w510) -> (Variant=w500:variant)
        n248 = call-poly "que_enqueue_message.vi"("error in (no error)"=w501, "Message Data"=w500, "Message"="Logging stop", "Message Queue"=w502) -> ("error out"=w506:errorcluster, "dup Message Queue"=w505:refnum<queue>)  [unwired: 6 in]
      }
      frame "Logging stop" {
        w535 = 0  # int32
        n249 = Variant To Data(error in=w532, type=w535, Variant=w531) -> (data=w533:i32, error out=w529:errorcluster)
        n250 = local read "log?"() -> (w527:bool)
        n251 = case shown="True" w527 {
          tunnel: w528 -> [w539 w543]
          tunnel: [w538 w542] -> w526
          tunnel: [w539 w541] -> w525
          tunnel: w529 -> [w538 w540]
          frame False {
          }
          frame True {
            n252 = global read "global_var.vi" "GUI strings"() -> (w544:string[])
            n253 = call "status_string_format.vi"("color"=enum16{"Black", "Blue", "Red", "Time"}."Time", "error in (no error)"=w540, "index"=55, "gui_strings"=w544, "Message Queue"=w543) -> ("error out"=w542:errorcluster, "dup Message Queue"=w541:refnum<queue>)  [unwired: 5 in]
          }
        }
        n254 = To Variant(anything=w533) -> (Variant=w534:variant)
        n255 = call-poly "que_enqueue_message.vi"("error in (no error)"=w526, "Message Data"=w534, "Message"="Stop", "Message Queue"=w524) -> ("error out"=w530:errorcluster)  [unwired: 6 in, 1 out]
      }
      frame "Ack logging stop" {
        # "### Handles the message that Logging is stopped ###"
        n256 = Variant To Data(error in=w558, type=cluster{path[], "int32":i32} {[], "int32"=0} ("output cluster"), Variant=w560) -> (data=w554:cluster{path[], "int32":i32}, error out=w557:errorcluster)
        n257 = local write "logging?"(FALSE ("runBar1?")) -> ()
        n258 = Unbundle(w554) -> (w553:path[], "int32"=w552:i32)
        n259 = for {
          tunnel: w553 -> [w595] mode=indexing
          tunnel: w550 -> [w596]
          tunnel: [w594] -> w551
          tunnel: w557 -> [w593]
          n260 = Empty String/Path?(string/path=w595) -> (empty?=w597:bool)
          n261 = case shown="False" w597 {
            tunnel: w596 -> [w603 _]
            tunnel: w595 -> [w602 _]
            tunnel: [w599 w605] -> w594
            tunnel: w593 -> [w598 w605]
            frame False {
              n262 = global read "global_var.vi" "GUI strings"() -> (w604:string[])
              n263 = call "status_string_format.vi"("log_file"=w602, "color"=enum16{"Black", "Blue", "Red", "Time"}."Time", "error in (no error)"=w598, "index"=41, "gui_strings"=w604, "Message Queue"=w603) -> ("error out"=w599:errorcluster)  [unwired: 4 in, 1 out]
            }
            frame True {
            }
          }
        }
        n264 = case shown="6666" w552 {
          tunnel: w551 -> [w570 w575 w583 w589]
          tunnel: w550 -> [w569 w578 w586 w592]
          tunnel: [w568 w582 w585 w591] -> w549
          tunnel: [w562 w581 w584 w590] -> w548
          tunnel: w547 -> [w564 _ _ _]
          frame 6666 {
            w566 = TRUE ("Priority Message? (F)")
            n265 = call-poly "que_enqueue_message.vi"("Priority Message? (F)"=w566, "error in (no error)"=w570, "Message"="Exit", "Message Queue"=w569) -> ("error out"=w567:errorcluster, "dup Message Queue"=w568:refnum<queue>)  [unwired: 6 in]
            n266 = call-poly "que_enqueue_message.vi"("Priority Message? (F)"=w566, "error in (no error)"=w567, "Message"="Stop", "Message Queue"=w564) -> ("error out"=w563:errorcluster)  [unwired: 6 in, 1 out]
            n267 = call "mules_wait_w_error.vi"("error in (no error)"=w563, "milliseconds to wait"=u32 200) -> ("error out"=w562:errorcluster)  [unwired: 1 in]
          }
          frame 3 {
            n268 = local read "eeg_device"() -> (w573:T3)
            n269 = global read "global_var.vi" "GUI strings"() -> (w577:string[])
            n270 = call "status_string_format.vi"("eeg_device"=w573, "color"=enum16{"Black", "Blue", "Red", "Time"}."Time", "error in (no error)"=w575, "index"=56, "gui_strings"=w577, "Message Queue"=w578) -> ("error out"=w574:errorcluster, "dup Message Queue"=w580:refnum<queue>)  [unwired: 4 in]
            n271 = call-poly "que_enqueue_message.vi"("error in (no error)"=w574, "Message"="Wait for source", "Message Queue"=w580) -> ("error out"=w581:errorcluster, "dup Message Queue"=w582:refnum<queue>)  [unwired: 7 in]
          }
          frame 1, Default {
            n272 = call-poly "que_enqueue_message.vi"("error in (no error)"=w583, "Message"="Wait for source", "Message Queue"=w586) -> ("error out"=w584:errorcluster, "dup Message Queue"=w585:refnum<queue>)  [unwired: 7 in]
          }
          frame 66 {
            n273 = call-poly "que_enqueue_message.vi"("error in (no error)"=w589, "Message"="Server start", "Message Queue"=w592) -> ("error out"=w590:errorcluster, "dup Message Queue"=w591:refnum<queue>)  [unwired: 7 in]
          }
        }
      }
      frame "WriteConsole" {
        # "### Writes a text in the Console-like text box, each line have its own color  ###"
        n274 = Variant To Data(error in=w607, type="", Variant=w622) -> (data=w619:string)  [unwired: 1 out]
        n275 = Search/Split String(string=w619, offset (0)=1 ("length (rest)")) -> (substring before match=w617:string, match + rest of string=w616:string)  [unwired: 1 in, 1 out]
        n276 = case shown="\"T\"" w617 {
          tunnel: w616 -> [w639 w648 w654 w660]
          tunnel: cluster{"String":string, "Color Box":u32} {"String"="", "Color Box"=16860} ("Cluster") -> [w637 w646 w652 w658]
          tunnel: [w636 w645 w651 w657] -> w606
          frame "T" {
            w642 = TRUE ("time colon?")
            n277 = call "mules_date2string.vi"("time colon?"=w642, "seconds?"=w642) -> ("time_string"=w641:string)  [unwired: 7 in, 2 out]
            n278 = call <vilib>:"Space Constant.vi"() -> ("String"=w640:string)
            n279 = Concatenate Strings(w641, w640, w639, "\r\n") -> (w638:string)
            n280 = Bundle(cluster=w637, "String"=w638, "Color Box"=u32 16777222) -> (w636:cluster{"String":string, "Color Box":u32})
          }
          frame "B" {
            n281 = Concatenate Strings(w648, "\r\n") -> (w644:string)
            n282 = Bundle(cluster=w646, "String"=w644, "Color Box"=u32 16860) -> (w645:cluster{"String":string, "Color Box":u32})
          }
          frame "K", Default {
            n283 = Concatenate Strings(w654, "\r\n") -> (w650:string)
            n284 = Bundle(cluster=w652, "String"=w650, "Color Box"=u32 16777222) -> (w651:cluster{"String":string, "Color Box":u32})
          }
          frame "R" {
            n285 = Concatenate Strings(w660, "\r\n") -> (w656:string)
            n286 = Bundle(cluster=w658, "String"=w656, "Color Box"=u32 16711680) -> (w657:cluster{"String":string, "Color Box":u32})
          }
        }
        n287 = Build Array (concatenate)(w620, w606) -> (w613:cluster{"String":string, "Color Box":u32}[])
        n288 = for {
          tunnel: w613 -> [w633] mode=indexing
          tunnel: [w632] -> w612 mode=indexing
          tunnel: [w631] -> w609
          i -> [w631]
          n289 = Unbundle(w633) -> ("String"=w632:string)  [unwired: 1 out]
        }
        n290 = Concatenate Strings(w612) -> (w611:string)
        n291 = property on="log_box" class="Str"("Text.Text"=w611, "Text.Scroll Position"=w609) -> (error out=w610:errorcluster)  [unwired: 2 in, 1 out]
        n292 = for {
          tunnel: w613 -> [w629] mode=indexing
          shift-right: [w624] -> _
          shift-left: 0 -> [w626]
          shift-right: [w623] -> w608
          shift-left: w610 -> [w627]
          n293 = Unbundle(w629) -> ("String"=w630:string, "Color Box"=w628:u32)
          n294 = String Length(string=w630) -> (length=w625:i32)
          n295 = Add(x=w625, y=w626) -> (x+y=w624:i32)
          n296 = property on="log_box" class="Str"(error in=w627, "Text.Selection End"=w624, "Text.Selection Start"=w626, "Text.FontColor"=w628) -> (error out=w623:errorcluster)  [unwired: 1 in, 1 out]
        }
      }
      frame "Confirm quit" {
        n297 = local read "acquiring?"() -> (w668:bool)
        n298 = local read "logging?"() -> (w662:bool)
        n299 = local read "serving?"() -> (w661:bool)
        n300 = Compound Arithmetic op=OR(w662, w661, w668) -> (w667:bool)
        n301 = case shown="True" w667 {
          tunnel: [TRUE ("Priority Message? (F)") w677] -> w670
          frame False {
          }
          frame True {
            n302 = global read "global_var.vi" "GUI strings"() -> (w676:string[])
            n303 = Index Array(array=w676, index #1=42 ("index")) -> (element #1=w675:string, element #2=w674:string, element #3=w673:string)  [unwired: 2 in]
            n304 = Two Button Dialog(message=w675, 1:w673, 2:w674) -> (T button?=w677:bool)
          }
        }
        n305 = case shown="True" w670 {
          tunnel: w663 -> [w678 w683]
          tunnel: w666 -> [w679 w682]
          tunnel: [w679 w681] -> w665
          tunnel: [w678 w680] -> w664
          frame False {
          }
          frame True {
            n306 = call-poly "que_enqueue_message.vi"("Priority Message? (F)"=TRUE, "error in (no error)"=w682, "Message"="Exit", "Message Queue"=w683) -> ("error out"=w681:errorcluster, "dup Message Queue"=w680:refnum<queue>)  [unwired: 6 in]
          }
        }
      }
      frame "Error", Default {
        # "### If there is an Error in any case, shows it and send Command Exit ###"
        n307 = Variant To Data(error in=w693, type=errorcluster {"status"=FALSE, "code"=0, "source"=""} ("error constant"), Variant=w692) -> (data=w698:errorcluster, error out=w688:errorcluster)
        n308 = call <vilib>:"Simple Error Handler.vi"("error in (no error)"=w698) -> ()  [unwired: 4 in, 5 out]
        n309 = call-poly "que_enqueue_message.vi"("Priority Message? (F)"=TRUE, "Message"="Exit", "Message Queue"=w691) -> ("error out"=w696:errorcluster, "dup Message Queue"=w686:refnum<queue>)  [unwired: 7 in]
        n310 = call <vilib>:"Clear Errors.vi"("error in (no error)"=w688) -> ("error out"=w687:errorcluster)  [unwired: 6 in]
        n311 = Merge Errors(w696, w687) -> (w690:errorcluster)
      }
      frame "Exit" {
        w699 = TRUE ("Priority Message? (F)")
        # "Stops while of UI Message Loop"
        # "Send Exit Message to Loops:\n-Acquisition\n-Server\n-Logging"
        # "Send Stop Event [0]"
        # "Destroy ALL ques"
        n312 = call "uev_fire_user_event_stop.vi"("User Event - Stop"=w713) -> ()  [unwired: 10 in, 1 out]
        n313 = Release Queue(queue=w715, error in (no error)=w714) -> (error out=w709:errorcluster)  [unwired: 1 in, 2 out]
        n314 = Release Queue(queue=w708, error in (no error)=w709) -> (error out=w706:errorcluster)  [unwired: 1 in, 2 out]
        n315 = call-poly "que_enqueue_message.vi"("Priority Message? (F)"=w699, "Message"=w702, "Message Queue"=w711) -> ()  [unwired: 7 in, 2 out]
        n316 = call-poly "que_enqueue_message.vi"("Priority Message? (F)"=w699, "Message"=w702, "Message Queue"=w712) -> ()  [unwired: 7 in, 2 out]
        n317 = call-poly "que_enqueue_message.vi"("Priority Message? (F)"=w699, "Message"=w702, "Message Queue"=w701) -> ()  [unwired: 7 in, 2 out]
        n318 = Release Queue(queue=w707, error in (no error)=w706) -> (error out=w705:errorcluster)  [unwired: 1 in, 2 out]
        n319 = Release Queue(queue=w704, error in (no error)=w705) -> (error out=w703:errorcluster)  [unwired: 1 in, 2 out]
        n320 = Stop(stop? (T)=w699) -> ()
      }
    }
    n321 = call "uev_error_handler_message_handling_loop.vi"("error in (no error)"=w64, "Message Queue"=w53) -> ("dup error in"=w56:errorcluster)  [unwired: 8 in, 1 out]
  }
  n322 = while {
    shift-right: [w723] -> w38
    shift-left: w6 -> [w722]
    tunnel: w21 -> [w721]
    tunnel: [w717] -> w37
    tunnel: w3 -> [w716]
    stop <- w718 stop-if-true
    # "Event Handling Loop"
    n323 = event shown="[5] \"config_files\": Value Change" {
      selector: w722 -> [_ _ _ _ _ _ _ _]
      dyn-events: [_ _ _ _ _ _ _ _] -> w723
      timeout: _ -> [_ _ _ _ _ _ _ _]
      tunnel: w721 -> [_ w727 w744 w763 w792 w797 w803 w805]
      tunnel: [_ w726 w736 w762 w793 w798 w802 _] -> w720
      tunnel: [_ w725 w746 w761 w794 _ w801 _] -> w719
      tunnel: [TRUE ("Discard?") _ _ _ _ _ _ _] -> w718
      tunnel: w716 -> [_ _ w747 _ _ _ _ _]
      event User Event {
        # "Stops While of Event Handling Loop"
        n324 = event-data() -> ()  [unwired: 1 in, 4 out]
      }
      event "stop?": Value Change {
        n325 = event-data() -> ()  [unwired: 1 in, 2 out]
        n326 = case shown="True" "stop?" {
          tunnel: w727 -> [w729 w734]
          tunnel: [w729 w735] -> w726
          tunnel: [_ w732] -> w725
          frame False {
          }
          frame True {
            n327 = To Variant(anything=1) -> (Variant=w730:variant)
            n328 = call-poly "que_enqueue_message.vi"("Message Data"=w730, "Message"="Acquisition stop", "Message Queue"=w734) -> ("error out"=w732:errorcluster, "dup Message Queue"=w735:refnum<queue>)  [unwired: 7 in]
          }
        }
      }
      event Key Down {
        n329 = event-data() -> ("Char"=w745:i16)  [unwired: 1 in, 4 out]
        n330 = To Unsigned Byte Integer(number=w745) -> (unsigned 8bit integer=w741:u8)
        n331 = In Range and Coerce(upper limit=u8 57 ("Char"), x=w741, lower limit=u8 49 ("Char")) -> (In Range?=w738:bool)  [unwired: 1 out]
        n332 = Not(x=w738) -> (.not. x?=w740:bool)
        n333 = Or(x=w740, y="refuse mrk?") -> (x .or. y?=w737:bool)
        n334 = case shown="True" w737 {
          tunnel: w747 -> [w759 _]
          tunnel: [w756 _] -> w746
          tunnel: w741 -> [w755 _]
          tunnel: w744 -> [w753 w760]
          tunnel: [w750 w760] -> w736
          frame False {
            w757 = u8 0  # U8
            n335 = Type Cast(x=w755) -> (*(type *) &x=w752:string)  [unwired: 1 in]
            n336 = global read "global_var.vi" "GUI strings"() -> (w749:string[])
            n337 = Decimal String To Number(string=w752, default (0L)=w757) -> (number=w758:u8)  [unwired: 1 in, 1 out]
            n338 = call "status_string_format.vi"("marker"=w752, "color"=enum16{"Black", "Blue", "Red", "Time"}."Time", "index"=31, "gui_strings"=w749, "Message Queue"=w753) -> ("error out"=w751:errorcluster, "dup Message Queue"=w750:refnum<queue>)  [unwired: 5 in]
            n339 = Enqueue Element(queue=w759, element=w758, error in (no error)=w751) -> (error out=w756:errorcluster)  [unwired: 1 in, 2 out]
          }
          frame True {
          }
        }
      }
      event "log?", "tcp?": Value Change {
        n340 = event-data() -> ("CtlRef"=w765:refnum<vi>, "OldVal"=w764:bool)  [unwired: 1 in, 1 out]
        n341 = Or(x="log?", y="tcp?") -> (x .or. y?=w768:bool)
        n342 = case shown="False" w768 {
          tunnel: "log?" -> [_ w782]
          tunnel: "tcp?" -> [_ w781]
          tunnel: w765 -> [w771 _]
          tunnel: w764 -> [w770 _]
          tunnel: w763 -> [w769 w780]
          tunnel: [w769 w779] -> w762
          tunnel: [_ w778] -> w761
          frame False {
            n343 = global read "global_var.vi" "GUI strings"() -> (w774:string[])
            n344 = property class="Bool (strict)"(reference=w771, "Val(Sgnl)"=w770) -> ()  [unwired: 1 in, 2 out]
            n345 = Index Array(array=w774, index=32) -> (element=w773:string)
            n346 = One Button Dialog(message=w773) -> ()  [unwired: 1 in, 1 out]
          }
          frame True {
            n347 = Build Array(w782, w781) -> (w776:bool[])
            n348 = To Variant(anything=w776) -> (Variant=w775:variant)
            n349 = call-poly "que_enqueue_message.vi"("Message Data"=w775, "Message"="Update booleans", "Message Queue"=w780) -> ("error out"=w778:errorcluster, "dup Message Queue"=w779:refnum<queue>)  [unwired: 7 in]
          }
        }
      }
      event "eeg_txtbox": Value Change {
        n350 = event-data() -> ("NewVal"=w790:string)  [unwired: 1 in, 5 out]
        n351 = Decimal String To Number(string=w790) -> (number=w787:i32)  [unwired: 2 in, 1 out]
        n352 = Increment(x=w787) -> (x+1=w789:i32)
        n353 = To Long Integer(number=w789) -> (32bit integer=w786:i32)
        n354 = Bundle(w786, path "", FALSE) -> (w784:cluster{i32, path, bool})  [unwired: 1 in]
        n355 = To Variant(anything=w784) -> (Variant=w788:variant)
        n356 = call-poly "que_enqueue_message.vi"("Message Data"=w788, "Message"="Device selected", "Message Queue"=w792) -> ("error out"=w794:errorcluster, "dup Message Queue"=w793:refnum<queue>)  [unwired: 7 in]
      }
      event "config_files": Value Change {
        n357 = event-data() -> ("NewVal"=w795:string)  [unwired: 1 in, 5 out]
        n358 = call-poly "que_enqueue_message.vi"("Message Data"=w795, "Message"="Read config", "Message Queue"=w797) -> ("dup Message Queue"=w798:refnum<queue>)  [unwired: 7 in, 1 out]
      }
      event "play?": Value Change {
        n359 = event-data() -> ()  [unwired: 1 in, 1 out]
        n360 = Not(x="play?") -> ()  [unwired: 1 out]
        n361 = call-poly "que_enqueue_message.vi"("Message"="Acquisition start", "Message Queue"=w803) -> ("error out"=w801:errorcluster, "dup Message Queue"=w802:refnum<queue>)  [unwired: 8 in]
      }
      event Panel Close? {
        # "Check if something is running, if not, just exit"
        n362 = event-data() -> ()  [unwired: 1 in, 1 out]
        n363 = call-poly "que_enqueue_message.vi"("Priority Message? (F)"=TRUE, "Message"="Confirm quit", "Message Queue"=w805) -> ()  [unwired: 7 in, 2 out]
        n364 = event-data("Discard?"=TRUE) -> ()  [unwired: 1 in, 1 out]
      }
    }
    n365 = call "uev_error_handler_event_loop.vi"("error in (no error)"=w719, "Message Queue"=w720) -> ("dup error in"=w717:errorcluster)  [unwired: 8 in, 1 out]
  }
  n366 = call "log_loop.vi"("Log queue"=w4, "Message Queues"=w2) -> ("error out"=w15:errorcluster)  [unwired: 9 in]
  n367 = while {
    shift-right: [w812] -> _
    shift-left: 0 ("y") -> [w814]
    tunnel: w6 -> [_]
    stop <- w809 stop-if-true
    # "Server Bar"
    n368 = Wait (ms)(milliseconds to wait=u32 50 ("millisecond multiple")) -> ()  [unwired: 1 out]
    n369 = Increment(x=w814) -> (x+1=w813:i32)
    n370 = Quotient & Remainder(x=w814, y=100) -> (x-y*floor(x/y)=w816:i32)  [unwired: 1 out]
    n371 = local read "stopBars"() -> (w809:bool)
    n372 = Add(x=w816, y=u32 10 ("millisecond multiple")) -> (x+y=w819:u32)
    n373 = Select(t=w813, s="serving?", f=0 ("y")) -> (s? t:f=w812:i32)
    n374 = Bundle(w816, w819) -> (→"srv_bar":cluster{i32, u32})  [unwired: 1 in]
  }
  n375 = while {
    shift-right: [w825] -> _
    shift-left: 0 ("y") -> [w827]
    tunnel: [w821] -> _
    tunnel: w6 -> [w821]
    stop <- w822 stop-if-true
    # "Logging Bar"
    n376 = Wait (ms)(milliseconds to wait=u32 50 ("millisecond multiple")) -> ()  [unwired: 1 out]
    n377 = Increment(x=w827) -> (x+1=w826:i32)
    n378 = Quotient & Remainder(x=w827, y=100) -> (x-y*floor(x/y)=w829:i32)  [unwired: 1 out]
    n379 = local read "stopBars"() -> (w822:bool)
    n380 = Add(x=w829, y=u32 10 ("millisecond multiple")) -> (x+y=w832:u32)
    n381 = Select(t=w826, s="logging?", f=0 ("y")) -> (s? t:f=w825:i32)
    n382 = Bundle(w829, w832) -> (→"log_bar":cluster{i32, u32})  [unwired: 1 in]
  }
  n383 = Unregister For Events(event registration refnum=w38, error in=w37) -> (error out=w36:errorcluster)
  n384 = Merge Errors(w36, w34, w24, w19, w15) -> (w35:errorcluster)
  n385 = call "uev_destroy_user_event_stop.vi"("error in (no error)"=w35, "User Event - Stop"=w33) -> ("error out"=w23:errorcluster)  [unwired: 9 in]
  n386 = Select(t=w22, s=w23, f=w22) -> (s? t:f=w7:bool)
  n387 = local write "stopBars"(w7) -> ()
  n388 = call "mules_exit_exe.vi"("Quit? (T)"=w7) -> ()  [unwired: 2 in]
